vi "Enable Source Output State.vi"(8 "error in":errorcluster, 10 "State":bool, 11 "VISA resource name":refnum<visa-resource-name>) -> (0 "error out":errorcluster, 3 "VISA resource name out":refnum<visa-resource-name>)   [LabVIEW 2015, in "IT-M3900C.lvlib"]
doc: "This command is used to enable or disable output.\n<b>State</b>\n0:Close the State\n1:Open the state"
uses:
  <instrlib>/IT-M3900C/IT-M3900C.lvlib
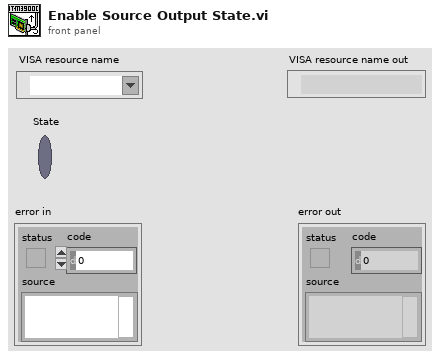
[diagram p1: front panel]
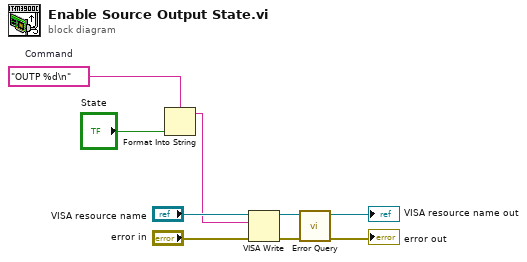
[diagram p0: block diagram]
diagram:
  w3 = "OUTP %d\n"  # Command
  n1 = Format Into String(format string=w3, "State") -> (resulting string=w1:string)  [unwired: 2 in, 1 out]
  n2 = VISA Write(VISA resource name="VISA resource name", write buffer=w1, error in (no error)="error in") -> (VISA resource name out=w6:refnum<visa-resource-name>, error out=w7:errorcluster)  [unwired: 1 out]
  n3 = call <instrlib>:"Error Query.vi"("error in"=w7, "VISA resource name"=w6) -> ("error out"=→"error out":errorcluster, "VISA resource name out"=→"VISA resource name out":refnum<visa-resource-name>)  [unwired: 6 in, 2 out]
